vi "music (old).vi"(7 "samples num":u32=1000, 9 "freq":dbl, 10 "packet valid":bool, 11 "fpga cluster":T1 {"Daughterboard Clock Rate" format="%#.3pHz"; "FPGA Data Clock Rate" format="%#.3pHz"; "Data Clock Rate" format="%#.3pHz"; "Characterization Data"."Frequencies [Hz]" format="%#_6p"; "EEPROM Characterization Header"."Pointer to Device Data Header" format="%x"; "EEPROM Characterization Header"."Checksum" format="%x"; "Device Data Header"."Pointer to Characterization Data" format="%x"; "Device Data Header"."Checksum" format="%x"; "EEPROM Header"."Pointer to User Header" format="%x"; "EEPROM Header"."Pointer to Factory Header" format="%x"; "EEPROM Header"."Product Code" format="%x"; "EEPROM Header"."Checksum" format="%x"}) -> (1 "max":dbl, 2 "spectrum":cluster{dbl[], dbl[]}(graph), 3 "Elements Remaining":u32)   [LabVIEW 2020]
uses:
  <instrlib>/niUsrpRio/Config/v1/Host/Public/niUsrpRio Session.ctl
  <instrlib>/_niInstr/Register Bus/v0/Host/Public/Register Bus Session.ctl
  <instrlib>/_niInstr/Register Bus/v0/Host/Private/Session Data.ctl
  <instrlib>/niUsrpRio/Config/v1/Host/Private/DB Queue Reference.ctl
  <instrlib>/niUsrpRio/Config/v1/Host/Private/Daughterboard Data.ctl
  <instrlib>/niUsrpRio/Config/v1/Host/Private/ATR state data.ctl
  <instrlib>/niUsrpRio/Config/v1/Host/Private/Antenna Configuration.ctl
  <instrlib>/niUsrpRio/Config/v1/Host/Private/CPLD Power Mode.ctl
  <instrlib>/niUsrpRio/Config/v1/Host/Public/EEPROM Header.ctl
  <instrlib>/niUsrpRio/Config/v1/Host/Public/EEPROM Device Data Header.ctl
  <instrlib>/niUsrpRio/Config/v1/Host/Public/EEPROM Characterization Header.ctl
  <instrlib>/niUsrpRio/Config/v1/Host/Public/Characterization Data.ctl
  <instrlib>/niUsrpRio/Config/v1/Host/Public/IQ Imbalance.ctl
  Host/SubVIs/Streaming Xvcr FPGA Ref.ctl
  <vilib>/Utility/error.llb/Error Cluster From Error Code.vi
  <vilib>/rvi/errors/niLvFpgaAdjustHostInterfaceError.vi
  <vilib>/rvi/interface/nirviMethod/nirviMethod.xnode
  <vilib>/rvi/errors/niLvFpgaMergeErrorWithErrorCode.vi
  <vilib>/FPGAPlugInAG/Dynamic/niLvFpga_ReadFifo_Dynamic.vi
  <instrlib>/_niInstr/Register Bus/v0/Host/niInstr Register Bus v0 Host.lvlib
  <instrlib>/niUsrpRio/Config/v1/Host/niUsrpRio Config v1 Host.lvlib
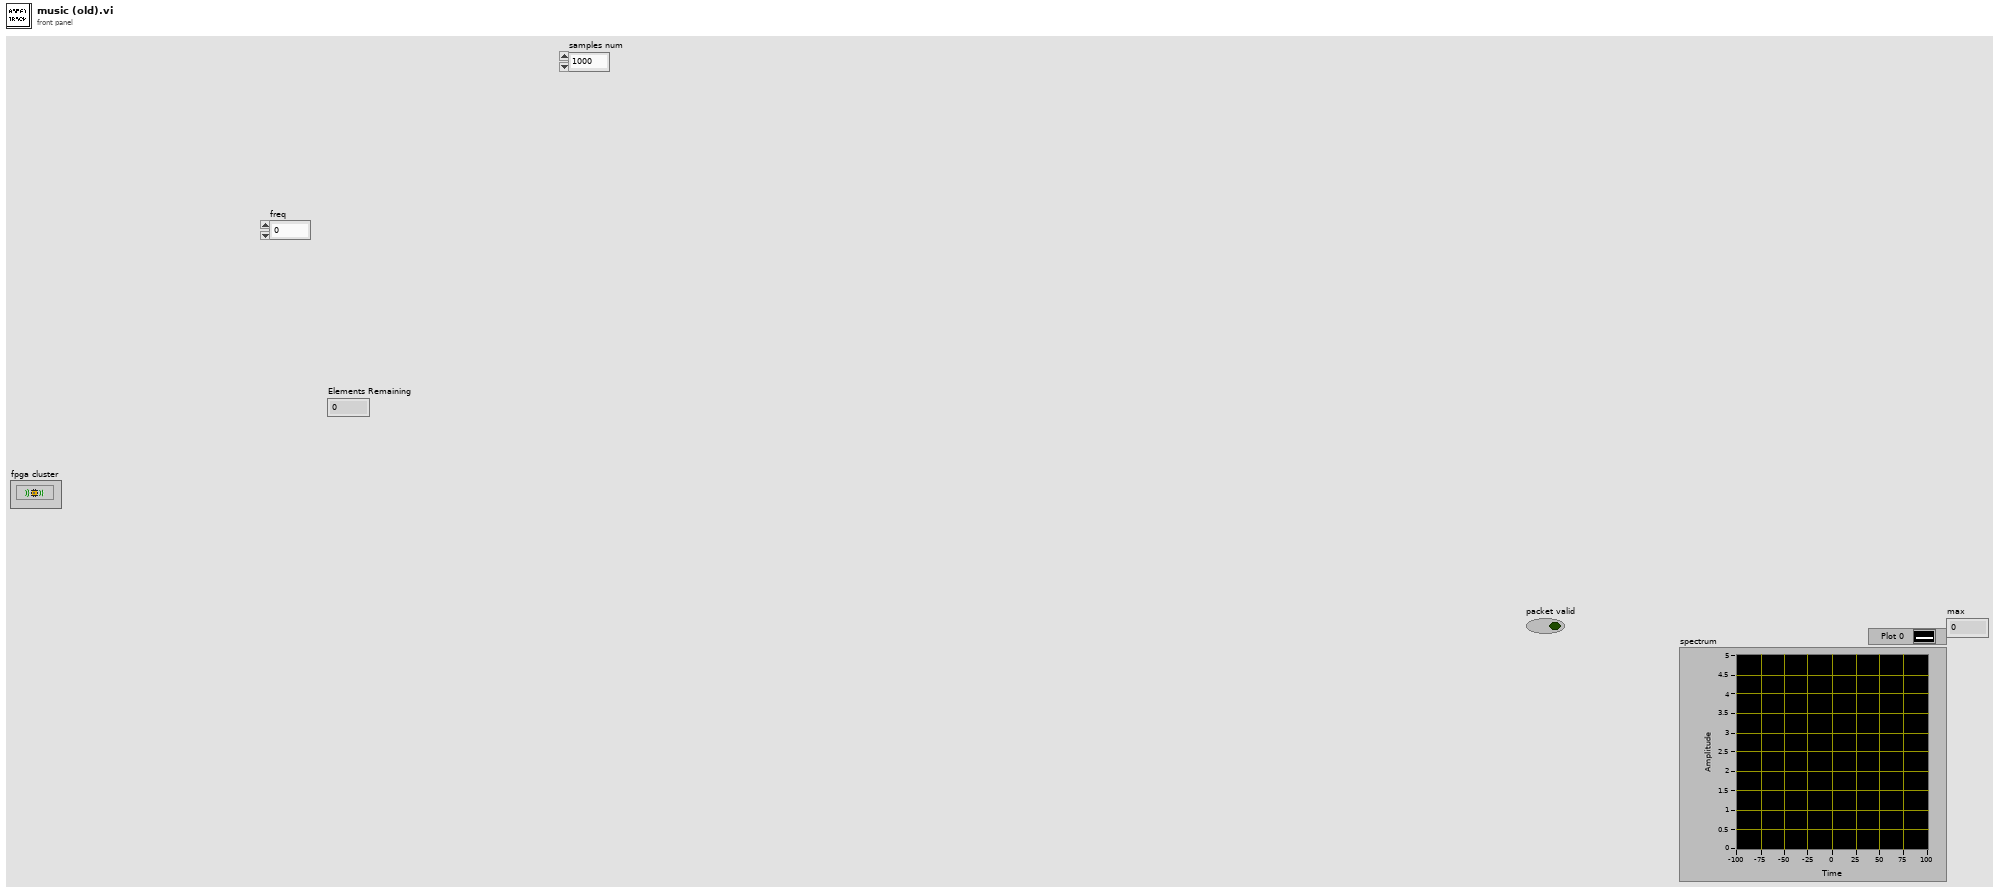
[diagram p1: front panel]
types:
  T1 = typedef "niUsrpRio Config v1 Host.lvlib/niUsrpRio Session.ctl" = cluster{"FPGA Interface":refnum<k20>, "RIO Interface Number":u32, "Data Clock Rate":u32, "FPGA Data Clock Rate":u32, "Global Settings Register Bus":T2, "Radio 0 Settings Register Bus":T2, "Radio 1 Settings Register Bus":T2, "Radio Settings Bus Semaphore":T3, "DB Queues":T4[], "Characterization Data Valid?":bool, "EEPROM Header":T5, "Device Data Header":T6, "EEPROM Characterization Header":T7, "Characterization Data":T8[], "FPGA Current Version":u32, "FPGA Oldest Compatible Version":u32, "Fixed Logic Current Version":u32, "Fixed Logic Oldest Compatible Version":u32, "FPGA Radio Settings Bus Current Version":u32, "FPGA Radio Settings Bus Oldest Compatible Version":u32, "FPGA Board Config Current Version":u32, "FPGA Board Config Oldest Compatible Version":u32, "Daughterboard Clock Rate":u32, "daughterboard configuration session handles":u64[]}
  T2 = typedef "niInstr Register Bus v0 Host.lvlib/Register Bus Session.ctl" = refnum<queue>
  T3 = typedef "Semaphore RefNum" = refnum<k1>
  T4 = typedef "niUsrpRio Config v1 Host.lvlib/DB Queue Reference.ctl" = refnum<queue>
  T5 = typedef "niUsrpRio Config v1 Host.lvlib/EEPROM Header.ctl" = cluster{"Checksum":u32, "Product Code":u16, "Hardware Current Version":u16, "Hardware Oldest Compatible Version":u16, "EEPROM Map Current Version":u16, "EEPROM Map Oldest Compatible Version":u16, "User Password":string, "Pointer to Factory Header":u32, "Pointer to User Header":u32, "Recommended Interval":u16, "Number of Reserved Bytes":i32, "Number of Daughterboards":u8, "Daughterboard IDs":u16[], "Daughterboard Serial Numbers":string[]}
  T6 = typedef "niUsrpRio Config v1 Host.lvlib/EEPROM Device Data Header.ctl" = cluster{"Checksum":u32, "Number of Channels":u8, "Number of Gain Settings":u16[], "Pointer to Characterization Data":u32[], "Number of Reserved Bytes":i32, "Number of Frequencies":u16[]}
  T7 = typedef "niUsrpRio Config v1 Host.lvlib/EEPROM Characterization Header.ctl" = cluster{"Checksum":u32, "Date":timestamp, "Temperature":sgl, "Misc. Info":string, "Pointer to Device Data Header":u32, "Number of Reserved Bytes":i32}
  T8 = typedef "niUsrpRio Config v1 Host.lvlib/Characterization Data.ctl" = cluster{"Gains[dB]":dbl[], "Frequencies [Hz]":dbl[], "IQ Imbalance Table":T9[], "Measured Gains[dB]":dbl[][]}
  T9 = typedef "niUsrpRio Config v1 Host.lvlib/IQ Imbalance.ctl" = cluster{"Gain Imbalance [linear]":dbl, "Phase Imbalance [radians]":dbl, "Offset":cdb}
  T10 = typedef "Streaming Xvcr FPGA Ref.ctl" = refnum<k20>
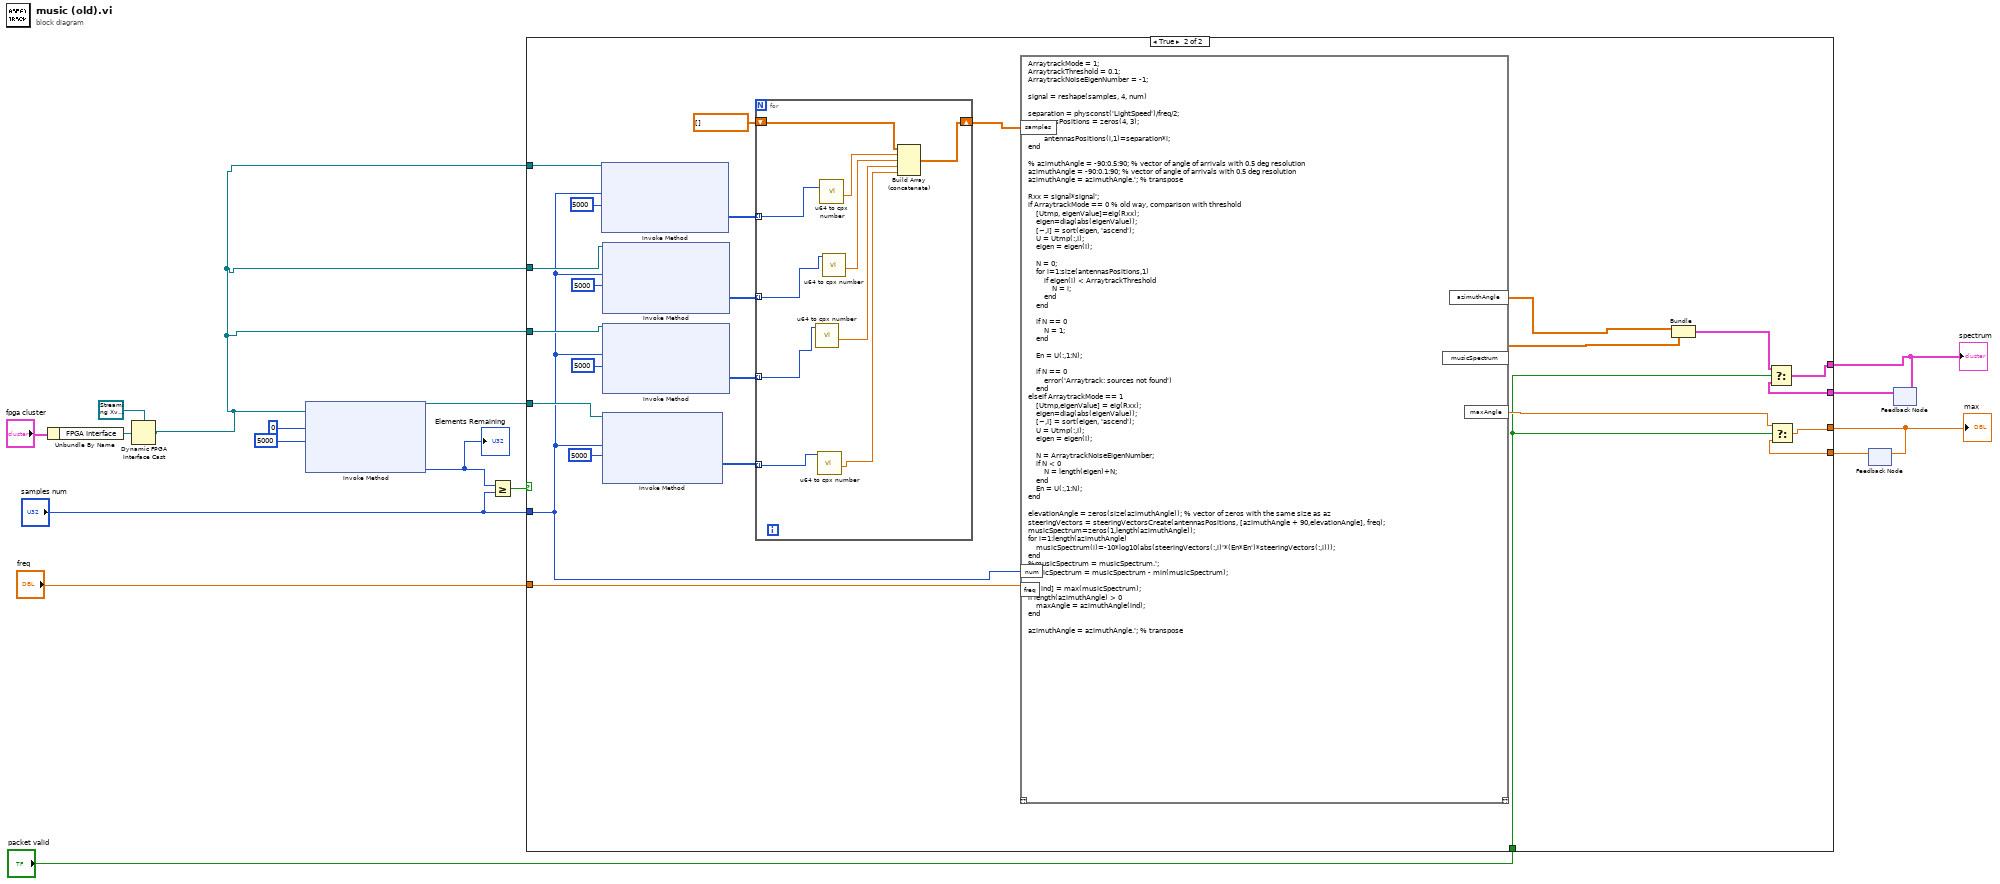
[diagram p0: block diagram]
diagram:
  n1 = Unbundle By Name("fpga cluster") -> ("FPGA Interface"=w13:refnum<k20>)
  n2 = Dynamic FPGA Interface Cast(Session In=T10 refnum ("Type"), Type=w13) -> (Session Out=w2:T10)
  n3 = xnode "Invoke Method"("FPGA VI Reference In"=w2, "Number of Elements"=u32 0, "Timeout (ms)"=5000) -> ("FPGA VI Reference Out"=w16:T10, "Elements Remaining"=w7:u32)  [unwired: 1 in, 2 out]
  "Elements Remaining" <- w7
  n4 = Greater Or Equal?(x=w7, y="samples num") -> (x >= y?=w10:bool)
  n5 = feedback #1() -> (w3:dbl)  [unwired: 1 in]
  n6 = feedback #2() -> (w5:cluster{dbl[], dbl[]})  [unwired: 1 in]
  n7 = case shown="True" w10 {
    tunnel: w16 -> [_ w43]
    tunnel: w2 -> [_ w37]
    tunnel: w2 -> [_ w36]
    tunnel: w2 -> [_ w35]
    tunnel: "samples num" -> [_ w31]
    tunnel: "freq" -> [_ w28]
    tunnel: [w18 w21] -> w6
    tunnel: w5 -> [w18 w20]
    tunnel: [w17 w24] -> w4
    tunnel: w3 -> [w17 w23]
    tunnel: "packet valid" -> [_ w19]
    frame False {
    }
    frame True {
      n8 = xnode "Invoke Method"("FPGA VI Reference In"=w37, "Number of Elements"=w31, "Timeout (ms)"=5000) -> ("Data"=w34:u64[])  [unwired: 1 in, 3 out]
      n9 = xnode "Invoke Method"("FPGA VI Reference In"=w43, "Number of Elements"=w31, "Timeout (ms)"=5000) -> ("Data"=w42:u64[])  [unwired: 1 in, 3 out]
      n10 = xnode "Invoke Method"("FPGA VI Reference In"=w36, "Number of Elements"=w31, "Timeout (ms)"=5000) -> ("Data"=w33:u64[])  [unwired: 1 in, 3 out]
      n11 = xnode "Invoke Method"("FPGA VI Reference In"=w35, "Number of Elements"=w31, "Timeout (ms)"=5000) -> ("Data"=w32:u64[])  [unwired: 1 in, 3 out]
      n12 = for {
        tunnel: w42 -> [w49] mode=indexing
        shift-right: [w51] -> w30
        shift-left: cdb[] [] -> [w52]
        tunnel: w34 -> [w53] mode=indexing
        tunnel: w33 -> [w47] mode=indexing
        tunnel: w32 -> [w48] mode=indexing
        n13 = call "u64 to cpx number.vi"("Numeric"=w48) -> ("x + iy"=w45:cdb)  [unwired: 10 in]
        n14 = call "u64 to cpx number.vi"("Numeric"=w49) -> ("x + iy"=w44:cdb)  [unwired: 10 in]
        n15 = call "u64 to cpx number.vi"("Numeric"=w53) -> ("x + iy"=w50:cdb)  [unwired: 10 in]
        n16 = call "u64 to cpx number.vi"("Numeric"=w47) -> ("x + iy"=w46:cdb)  [unwired: 10 in]
        n17 = Build Array (concatenate)(w52, w50, w46, w45, w44) -> (w51:cdb[])
      }
      n18 = script code="ArraytrackMode = 1;\nArraytrackThreshold = 0.1;\nArraytrackNoiseEigenNumber = -1;\n\nsignal = reshape(samples, 4, num)\n\nseparation = physconst('LightSpeed')/freq/2;\nantennasPositions = zeros(4, 3);\nfor i=1:4\n        antennasPositions(i,1)=separation*i;\nend\n\n% azimuthAngle = -90:0.5:90; % vector of angle of arrivals with 0.5 deg resolution\nazimuthAngle = -90:0.1:90; % vector of angle of arrivals with 0.5 deg resolution\nazimuthAngle = azimuthAngle.'; % transpose\n\nRxx = signal*signal';\nif ArraytrackMode == 0 % old way, comparison with threshold\n    [Utmp, eigenValue]=eig(Rxx);\n    eigen=diag(abs(eigenValue));\n    [~,I] = sort(eigen, 'ascend');\n    U = Utmp(:,I);\n    eigen = eigen(I);\n    \n    N = 0;\n    for i=1:size(antennasPositions,1)\n        if eigen(i) < ArraytrackThreshold\n            N = i;\n        end\n    end\n    \n    if N == 0\n        N = 1;\n    end\n    \n    En = U(:,1:N);\n    \n    if N == 0\n        error('Arraytrack: sources not found')\n    end\nelseif ArraytrackMode == 1\n    [Utmp,eigenValue] = eig(Rxx);\n    eigen=diag(abs(eigenValue));\n    [~,I] = sort(eigen, 'ascend');\n    U = Utmp(:,I);\n    eigen = eigen(I);\n    \n    N = ArraytrackNoiseEigenNumber;\n    if N < 0\n        N = length(eigen)+N;\n    end\n    En = U(:,1:N);\nend\n\nelevationAngle = zeros(size(azimuthAngle)); % vector of zeros with the same size as az\nsteeringVectors = steeringVectorsCreate(antennasPositions, [azimuthAngle + 90,elevationAngle], freq);\nmusicSpectrum=zeros(1,length(azimuthAngle));\nfor i=1:length(azimuthAngle)\n    musicSpectrum(i)=-10*log10(abs(steeringVectors(:,i)'*(En*En')*steeringVectors(:,i)));\nend\n%musicSpectrum = musicSpectrum.';\nmusicSpectrum = musicSpectrum - min(musicSpectrum);\n\n[~, ind] = max(musicSpectrum);\nif length(azimuthAngle) > 0\n    maxAngle = azimuthAngle(ind);\nend\n\nazimuthAngle = azimuthAngle.'; % transpose"("samples"=w30, "num"=w31, "freq"=w28) -> ("musicSpectrum"=w26:dbl[], "azimuthAngle"=w27:dbl[], "maxAngle"=w25:dbl)  [unwired: 1 in, 1 out]
      n19 = Bundle(w27, w26) -> (w22:cluster{dbl[], dbl[]})  [unwired: 1 in]
      n20 = Select(t=w22, s=w19, f=w20) -> (s? t:f=w21:cluster{dbl[], dbl[]})
      n21 = Select(t=w25, s=w19, f=w23) -> (s? t:f=w24:dbl)
    }
  }
  "spectrum" <- w6
  "max" <- w4
  n22 = feedback-in #1(w4) -> ()
  n23 = feedback-in #2(w6) -> ()
